vi "Parse qUSG PAM Answer.vi"(0 "Answer To Parse":string, 5 "error in":errorcluster) -> (14 "Array of ParametersInfo":T1[](array[typedef]), 19 "error out":errorcluster)   [LabVIEW 2026]
doc: "Parse a SPV? structured answer to a array of parameter sets.\nWill return a warning if some parameters could not be parsed."
uses:
  GeneralCommands/ParameterInfoSet.ctl
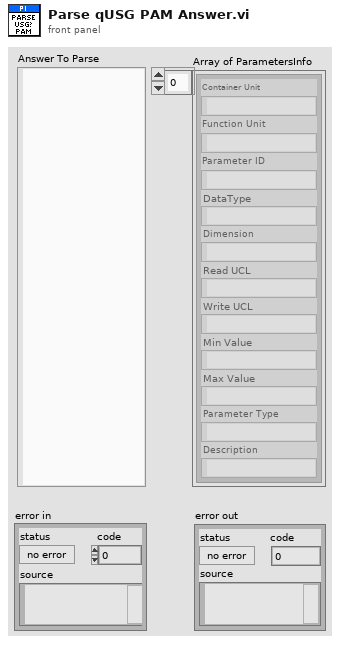
[diagram p1: front panel]
types:
  T1 = typedef "ParameterInfoSet.ctl" = cluster{"Container Unit":string, "Function Unit":string, "Parameter ID":string, "DataType":string, "Dimension":string, "Read UCL":string, "Write UCL":string, "Min Value":string, "Max Value":string, "Parameter Type":string, "Description":string}
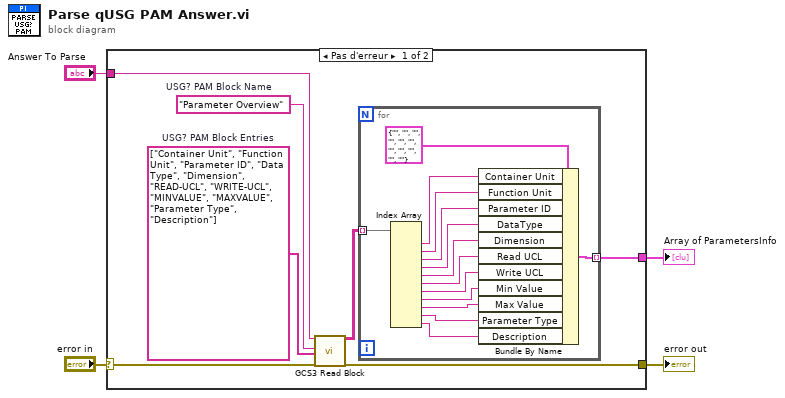
[diagram p0: block diagram]
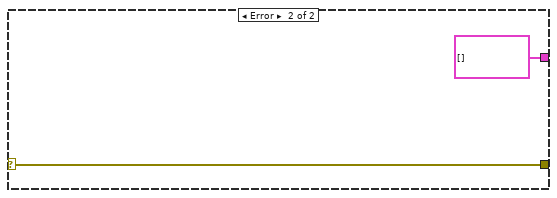
[diagram p2: hidden frame]
diagram:
  n1 = case shown="Pas d'erreur" "error in" {
    selector: "error in" -> [w11 w27]
    tunnel: "Answer To Parse" -> [w10 _]
    tunnel: [w5 T1[] []] -> w3
    tunnel: [w6 w27] -> w1
    frame No Error {
      w8 = string[] ["Container Unit", "Function Unit", "Parameter ID", "Data Type", "Dimension", "READ-UCL", "WRITE-UCL", "MINVALUE", "MAXVALUE", "Parameter Type", "Description"]  # USG? PAM Block Entries
      w9 = "Parameter Overview"  # USG? PAM Block Name
      n2 = call "GCS3 Read Block.vi"("GCS 3.0 Block to Parse"=w10, "Expected GCS 3.0 Block Name"=w9, "List of expected GCS 3.0 Block Entries"=w8, "error in"=w11) -> ("List of extracted GCS 3.0 Block Entries"=w7:string[][], "error out"=w6:errorcluster)  [unwired: 14 in]
      n3 = for {
        tunnel: w7 -> [w13] mode=indexing
        tunnel: [w12] -> w5 mode=indexing
        n4 = Index Array(array=w13) -> (element #1=w17:string, element #2=w14:string, element #3=w15:string, element #4=w16:string, element #5=w18:string, element #6=w19:string, element #7=w20:string, element #8=w21:string, element #9=w22:string, element #10=w23:string, element #11=w24:string)  [unwired: 11 in]
        n5 = Bundle By Name(cluster=T1 {"Container Unit"="", "Function Unit"="", "Parameter ID"="", "DataType"="", "Dimension"="", "Read UCL"="", "Write UCL"="", "Min Value"="", "Max Value"="", "Parameter Type"="", "Description"=""} ("ParameterInfoSet"), "Container Unit"=w17, "Function Unit"=w14, "Parameter ID"=w15, "DataType"=w16, "Dimension"=w18, "Read UCL"=w19, "Write UCL"=w20, "Min Value"=w21, "Max Value"=w22, "Parameter Type"=w23, "Description"=w24) -> (w12:T1)
      }
    }
    frame Error {
    }
  }
  "Array of ParametersInfo" <- w3
  "error out" <- w1
